vi "Read New Message Event.vi"(8 "error in (no error)":errorcluster, 11 "Pub Sub Event Channel in":refnum<class "Pub Sub Event Channel.lvclass">) -> (0 "error out":errorcluster, 2 "New Message Event":refnum<user-event>, 3 "Pub Sub Event Channel out":refnum<class "Pub Sub Event Channel.lvclass">)   [LabVIEW 2020, in "Actor Pub Sub Channels.lvlib" / "Pub Sub Event Channel.lvclass"]
uses:
  Pub Sub Event Channel.lvclass
  <vilib>/ActorFramework/Message/Message.lvclass
  Pub Sub Event Channel.lvclass/Pub Sub Event Channel.ctl
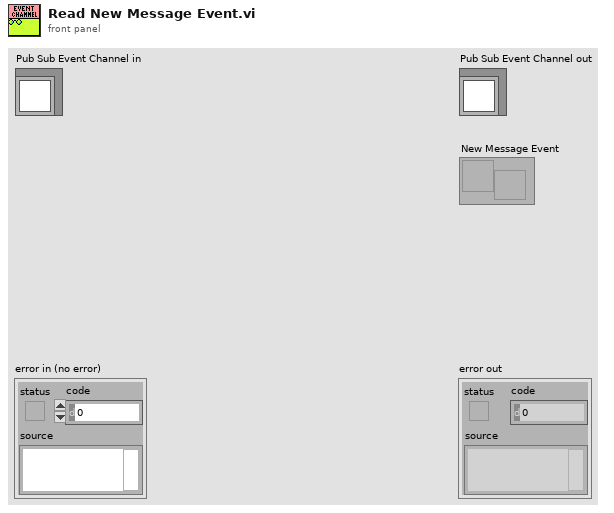
[diagram p1: front panel]
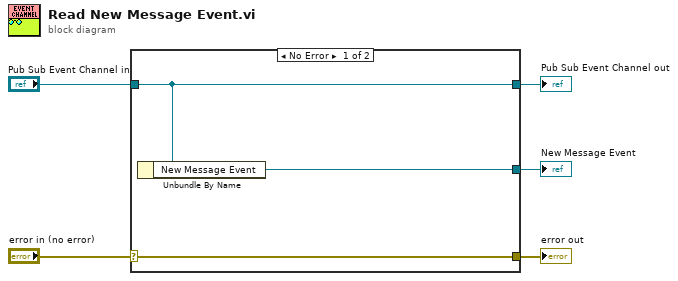
[diagram p0: block diagram]
diagram:
  n1 = case shown="No Error" "error in (no error)" {
    selector: "error in (no error)" -> [w8 w9]
    tunnel: [w8 w9] -> w4
    tunnel: [w7 w10] -> w2
    tunnel: "Pub Sub Event Channel in" -> [w7 w10]
    tunnel: [w6 _] -> w1
    frame No Error {
      n2 = Unbundle By Name(w7) -> ("New Message Event"=w6:refnum<user-event>)
    }
    frame Error {
    }
  }
  "error out" <- w4
  "Pub Sub Event Channel out" <- w2
  "New Message Event" <- w1
